vi "Release Priority Queue.vi"(8 "error in (no error)":errorcluster, 11 "Priority Message Queue in":refnum<class "Priority Message Queue.lvclass">) -> (0 "error out":errorcluster, 2 "Remaining Elements":refnum<class "Message.lvclass">[](array[class]))   [LabVIEW 2020, in "Artifex.lvlib" / "Priority Message Queue.lvclass"]
uses:
  Priority Message Queue.lvclass
  Message/Message.lvclass
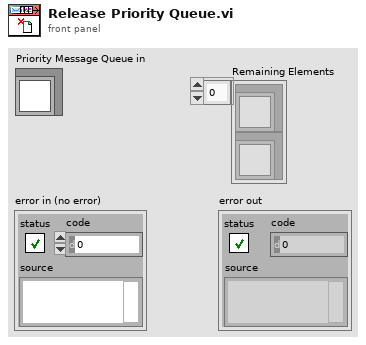
[diagram p1: front panel]
types:
  T1 = typedef "Artifex.lvlib/Priority Message Queue.lvclass/Ref Data.ctl" = cluster{"# Waiting":u32, "Buffers":refnum<queue>[], "Wait Msg":refnum<queue>, "Wait Prior":refnum<queue>}
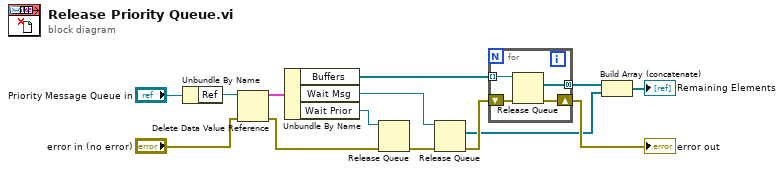
[diagram p0: block diagram]
diagram:
  n1 = Unbundle By Name("Priority Message Queue in") -> ("Ref"=w12:refnum<data-value>)
  n2 = Delete Data Value Reference(data value reference=w12, error in="error in (no error)") -> (data value=w11:T1, error out=w9:errorcluster)
  n3 = Unbundle By Name(w11) -> ("Buffers"=w5:refnum<queue>[], "Wait Msg"=w7:refnum<queue>, "Wait Prior"=w8:refnum<queue>)
  n4 = Release Queue(queue=w8, error in (no error)=w9) -> (error out=w6:errorcluster)  [unwired: 1 in, 2 out]
  n5 = Release Queue(queue=w7, error in (no error)=w6) -> (remaining elements=w2:refnum<class "Message.lvclass">[], error out=w4:errorcluster)  [unwired: 1 in, 1 out]
  n6 = for {
    tunnel: w5 -> [w18] mode=indexing
    shift-right: [w16] -> w14
    shift-left: w4 -> [w17]
    tunnel: [w15] -> w3 mode=concatenating
    n7 = Release Queue(queue=w18, error in (no error)=w17) -> (remaining elements=w15:refnum<class "Message.lvclass">[], error out=w16:errorcluster)  [unwired: 1 in, 1 out]
  }
  "error out" <- w14
  n8 = Build Array (concatenate)(w3, w2) -> (→"Remaining Elements":refnum<class "Message.lvclass">[])
